vi "fo_NewDicomFile.vi"(8 "error in (no error)":errorcluster, 11 "DICOM Info":path) -> (0 "error out":errorcluster, 3 "String":string)   [LabVIEW 2013, in "main.lvlib"]
uses:
  main.lvlib
  C:/Users/Simon/SkyDrive/LabView/2013/DM2020/bin/Dicom.dll
  bin/Dicom.dll
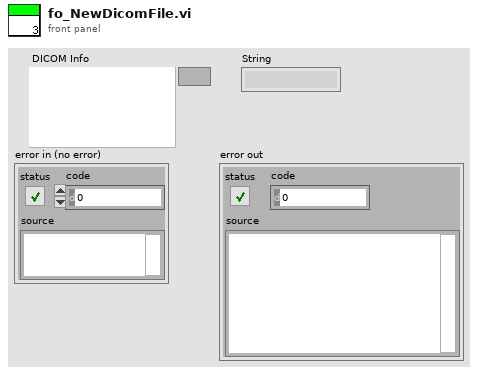
[diagram p1: front panel]
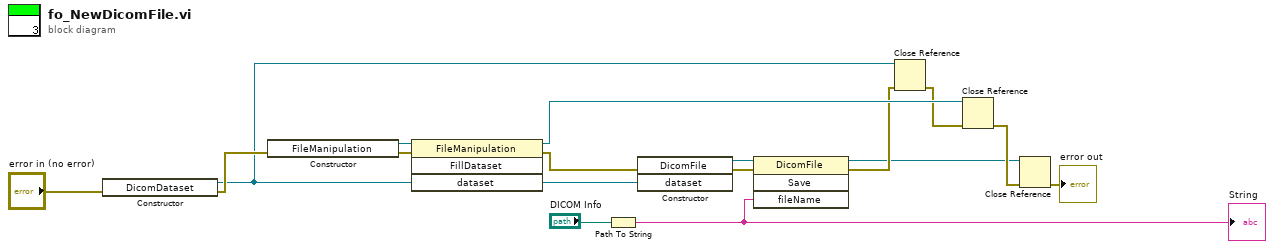
[diagram p0: block diagram]
diagram:
  n1 = constructor class="DicomDataset"(error in="error in (no error)") -> (reference out=w1:refnum<k24>, error out=w13:errorcluster)  [unwired: 2 in, 1 out]
  n2 = constructor class="FileManipulation"(error in=w13) -> (reference out=w7:refnum<k24>, error out=w12:errorcluster)  [unwired: 2 in, 1 out]
  n3 = invoke class="FileManipulation" method="FillDataset"(reference=w7, error in=w12, "dataset"=w1) -> (reference out=w15:refnum<k24>, error out=w14:errorcluster)  [unwired: 1 in, 2 out]
  n4 = Path To String(path="DICOM Info") -> (string=w16:string)
  "String" <- w16
  n5 = constructor class="DicomFile"(error in=w14, "dataset"=w1) -> (reference out=w8:refnum<k24>, error out=w9:errorcluster)  [unwired: 2 in, 2 out]
  n6 = invoke class="DicomFile" method="Save"(reference=w8, error in=w9, "fileName"=w16) -> (reference out=w5:refnum<k24>, error out=w10:errorcluster)  [unwired: 1 in, 2 out]
  n7 = Close Reference(reference=w1, error in (no error)=w10) -> (error out=w11:errorcluster)
  n8 = Close Reference(reference=w15, error in (no error)=w11) -> (error out=w6:errorcluster)
  n9 = Close Reference(reference=w5, error in (no error)=w6) -> (error out=→"error out":errorcluster)
